vi "setImageBinning.vi"(8 "error in (no error)":errorcluster, 10 "Image Binning":T1, 11 "CameraAcquisitor.lvclass in":refnum<class "CameraAcquisitor.lvclass">) -> (0 "error out":errorcluster, 3 "CameraAcquisitor.lvclass out":refnum<class "CameraAcquisitor.lvclass">)   [LabVIEW 2009, in "Hardware.lvlib" / "Channels.lvlib" / "CameraAcquisitor.lvclass"]
uses:
  CameraAcquisitor.lvclass
  CameraAcquisitor.lvclass/CameraAcquisitor.ctl
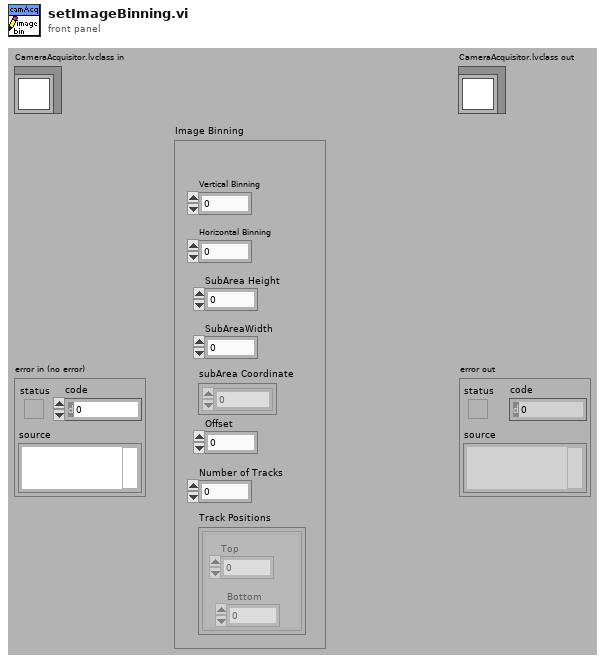
[diagram p1: front panel]
types:
  T1 = cluster{"Vertical Binning":dbl, "Horizontal Binning":dbl, "SubArea Height":dbl, "SubAreaWidth":dbl, "Offset":dbl, "Number of Tracks":dbl, "Track Positions":cluster{"Top":dbl, "Bottom ":dbl}[], "subArea Coordinate":dbl[]}
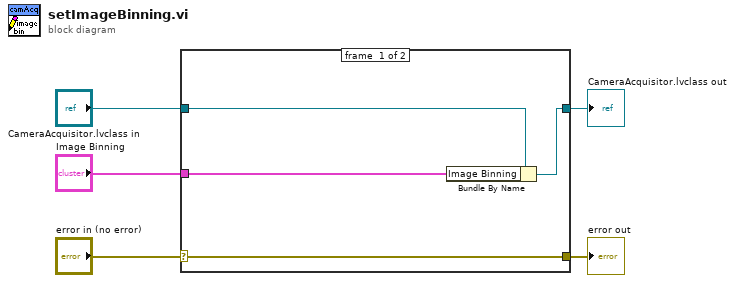
[diagram p0: block diagram]
diagram:
  n1 = case shown="No Error" "error in (no error)" {
    selector: "error in (no error)" -> [w9 w10]
    tunnel: [w9 w10] -> w4
    tunnel: [w7 w11] -> w2
    tunnel: "CameraAcquisitor.lvclass in" -> [w8 w11]
    tunnel: "Image Binning" -> [w6 _]
    frame #0 {
      n2 = Bundle By Name(cluster=w8, "Image Binning"=w6) -> (w7:refnum<class "CameraAcquisitor.lvclass">)
    }
    frame #1 {
    }
  }
  "error out" <- w4
  "CameraAcquisitor.lvclass out" <- w2
